vi "Size 2 Force Labels.vi"(3 "Size":T1) -> (0 "Actuator Space Labels":string[](array[string]), 1 "Cartesian Space Labels In":string[](array[string]))   [LabVIEW 2009]
uses:
  Data Access Objects/Metadata/LBCB Size.ctl
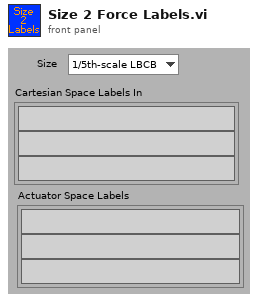
[diagram p1: front panel]
types:
  T1 = typedef "LBCB Size.ctl" = enum16{"1/5th-scale LBCB", "Full-scale LBCB", "Portable LBCB"}
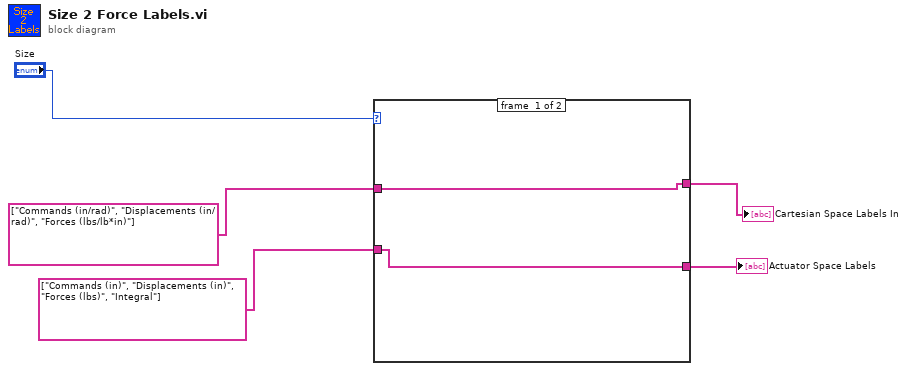
[diagram p0: block diagram]
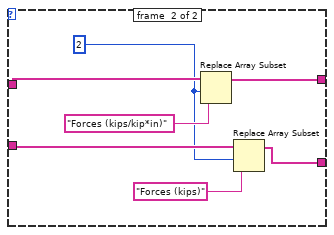
[diagram p2: hidden frame]
diagram:
  n1 = case shown="\"1/5th-scale LBCB\", Default" "Size" {
    tunnel: string[] ["Commands (in/rad)", "Displacements (in/rad)", "Forces (lbs/lb*in)"] ("Cartesian Space Labels") -> [w7 w14]
    tunnel: string[] ["Commands (in)", "Displacements (in)", "Forces (lbs)", "Integral"] ("Actuator Space Labels") -> [w6 w10]
    tunnel: [w7 w12] -> w2
    tunnel: [w6 w9] -> w1
    frame #0 {
    }
    frame #1 {
      w8 = 2 ("index")
      n2 = Replace Array Subset(array=w14, new element="Forces (kips/kip*in)" ("new element/subarray"), index=w8) -> (w12:string[])
      n3 = Replace Array Subset(array=w10, new element="Forces (kips)" ("new element/subarray"), index=w8) -> (w9:string[])
    }
  }
  "Actuator Space Labels" <- w1
  "Cartesian Space Labels In" <- w2
